vi "Configure Range Table (Spurious Emissions - Filter Type).vi"(0 "VISA resource name":refnum<visa-resource-name>, 5 "Filter Type List":i32[](array[ring])=[0, 0] items=["Gaussian (Normal)", "Flattop"], 11 "error in (no error)":errorcluster) -> (4 "VISA resource name out":refnum<visa-resource-name>, 15 "error out":errorcluster)   [LabVIEW 2014, in "Agilent MXA Series.lvlib"]
doc: "Configures the Filter Type settings under Range Table for Spurious Emissions measurement type."
uses:
  Agilent MXA Series.lvlib
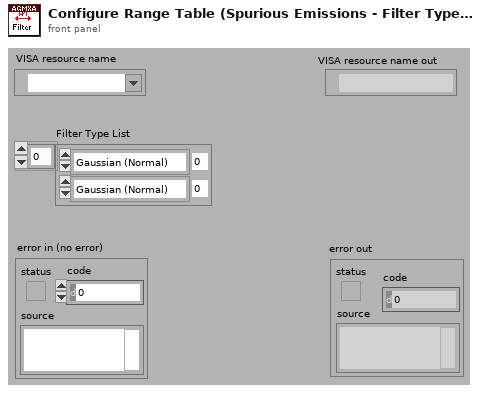
[diagram p1: front panel]
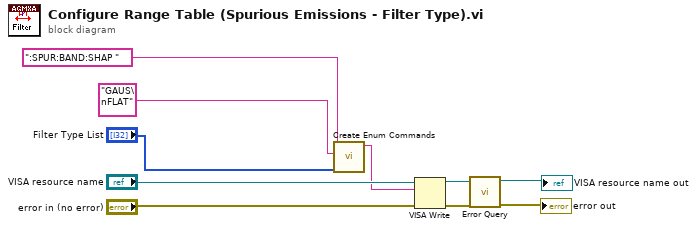
[diagram p0: block diagram]
diagram:
  n1 = call "Create Enum Commands.vi"("Enum Values"="Filter Type List", "Multi-line Text"="GAUS\nFLAT" ("multi-line string"), "Commands"=":SPUR:BAND:SHAP ") -> ("Result"=w1:string)  [unwired: 8 in]
  n2 = VISA Write(VISA resource name="VISA resource name", write buffer=w1, error in (no error)="error in (no error)") -> (VISA resource name out=w7:refnum<visa-resource-name>, error out=w8:errorcluster)  [unwired: 1 out]
  n3 = call "Error Query.vi"("error in (no error)"=w8, "VISA resource name"=w7) -> ("error out"=→"error out":errorcluster, "VISA resource name out"=→"VISA resource name out":refnum<visa-resource-name>)  [unwired: 6 in, 2 out]
